vi "log analysis_gps.vi"() -> ()   [LabVIEW 2019] (continued)
,37.37108222334,126.72339800305,8.3261,22.3000,-0.1005,0.2888,0.0175,-1.549699637,0.826090686,104.570528927,0.4090,0.2977,0.5394,0.1094,0.0929,0.0762,0.1525,0.1522,4.9251,0f000001,0*19ed46e2\n\t", "INSPVAXA,USB3,0,46.5,FINESTEERING,2107,281999.350,02000000,471d,15824;INS_ALIGNMENT_COMPLETE,INS_RTKFIXED,37.37108175635,126.72339952041,8.3297,22.3000,-0.1125,0.3020,0.0389,-1.388953063,0.939960250,105.504121807,0.4075,0.2973,0.5375,0.1091,0.0928,0.0761,0.1524,0.1521,4.9251,0f000001,0*0f043892\n\t", "INSPVAXA,USB3,0,46.5,FINESTEERING,2107,281999.850,02000000,471d,15824;INS_ALIGNMENT_COMPLETE,INS_RTKFIXED,37.37108126318,126.72340101598,8.3324,22.3000,-0.1208,0.2855,0.0176,-1.235609650,1.001617450,106.317928452,0.4075,0.2973,0.5375,0.1091,0.0928,0.0761,0.1524,0.1521,4.9251,0f000001,0*a366704e\n\t", "INSPVAXA,USB3,0,45.5,FINESTEERING,2107,282000.350,02000000,471d,15824;INS_ALIGNMENT_COMPLETE,INS_RTKFIXED,37.37108078810,126.72340249141,8.3350,22.3000,-0.1085,0.2765,0.0052,-1.369966017,1.132397768,106.939829870,0.4067,0.2969,0.5359,0.1090,0.0927,0.0761,0.1523,0.1521,4.9261,0f000001,0*76e4d7c9\n\t", "INSPVAXA,USB3,0,45.5,FINESTEERING,2107,282000.850,02000000,471d,15824;INS_ALIGNMENT_COMPLETE,INS_RTKFIXED,37.37108030098,126.72340396380,8.3376,22.3000,-0.1078,0.2732,0.0027,-1.376343983,1.101027936,107.303720735,0.4067,0.2969,0.5359,0.1090,0.0927,0.0761,0.1523,0.1521,4.9261,0f000001,0*d0ca4e8b\n\t", "INSPVAXA,USB3,0,48.0,FINESTEERING,2107,282001.350,02000000,471d,15824;INS_ALIGNMENT_COMPLETE,INS_RTKFIXED,37.37107981419,126.72340544381,8.3410,22.3000,-0.1015,0.2654,0.0098,-1.448342313,0.934631006,107.625890193,0.4067,0.2967,0.5346,0.1090,0.0928,0.0761,0.1522,0.1521,4.9276,0f000001,0*0452f07a\n\t", "INSPVAXA,USB3,0,48.0,FINESTEERING,2107,282001.850,02000000,471d,15824;INS_ALIGNMENT_COMPLETE,INS_RTKFIXED,37.37107932053,126.72340689230,8.3455,22.3000,-0.1081,0.2753,0.0156,-1.395073835,0.867862564,107.855111716,0.4067,0.2967,0.5346,0.1090,0.0928,0.0761,0.1522,0.1521,4.9276,0f000001,0*57502385\n\t", "INSPVAXA,USB3,0,47.5,FINESTEERING,2107,282003.350,02000000,471d,15824;INS_ALIGNMENT_COMPLETE,INS_RTKFIXED,37.37107789784,126.72341117734,8.3560,22.3000,-0.1094,0.2769,0.0199,-1.466008388,0.636532591,108.200024976,0.4065,0.2960,0.5312,0.1093,0.0930,0.0760,0.1520,0.1521,4.9306,0f000001,0*2f9a30b4\n\t", "INSPVAXA,USB3,0,47.5,FINESTEERING,2107,282003.850,02000000,471d,15824;INS_ALIGNMENT_COMPLETE,INS_RTKFIXED,37.37107739435,126.72341272898,8.3600,22.3000,-0.1006,0.2711,0.0114,-1.521008315,0.580444752,108.231718498,0.4065,0.2960,0.5312,0.1093,0.0930,0.0760,0.1520,0.1521,4.9306,0f000001,0*1b9fd745\n\t", "INSPVAXA,USB3,0,50.0,FINESTEERING,2107,282004.350,02000000,471d,15824;INS_ALIGNMENT_COMPLETE,INS_RTKFIXED,37.37107686919,126.72341426546,8.3651,22.3000,-0.1209,0.2828,0.0059,-1.390875360,0.569748446,108.156890117,0.4068,0.2963,0.5308,0.1095,0.0933,0.0761,0.1519,0.1521,4.9320,0f000001,0*3c184099\n\t", "INSPVAXA,USB3,0,51.0,FINESTEERING,2107,282005.850,02000000,471d,15824;INS_ALIGNMENT_COMPLETE,INS_RTKFIXED,37.37107540800,126.72341870261,8.3803,22.3000,-0.1004,0.2666,0.0170,-1.392102628,0.780129510,106.805722227,0.4082,0.2971,0.5322,0.1099,0.0935,0.0762,0.1518,0.1521,4.9335,0f000001,0*c4f2d669\n\t", "INSPVAXA,USB3,0,50.5,FINESTEERING,2107,282006.350,02000000,471d,15824;INS_ALIGNMENT_COMPLETE,INS_RTKFIXED,37.37107495980,126.72342017770,8.3861,22.3000,-0.1091,0.2763,0.0150,-1.313432371,0.996573808,106.046100672,0.4084,0.2972,0.5323,0.1099,0.0934,0.0763,0.1516,0.1520,4.9349,0f000001,0*72236ee9\n\t", "INSPVAXA,USB3,0,49.0,FINESTEERING,2107,282007.350,02000000,471d,15824;INS_ALIGNMENT_COMPLETE,INS_RTKFIXED,37.37107412137,126.72342315241,8.3985,22.3000,-0.0946,0.2769,0.0276,-1.358512110,1.052240106,104.351657391,0.4091,0.2973,0.5323,0.1098,0.0932,0.0763,0.1515,0.1519,4.9361,0f000001,0*6aff20b9\n\t", "INSPVAXA,USB3,0,47.0,FINESTEERING,2107,282009.350,02000000,471d,15824;INS_ALIGNMENT_COMPLETE,INS_RTKFIXED,37.37107260212,126.72342930936,8.4118,22.3000,-0.0884,0.2755,0.0223,-1.652819508,0.448050355,102.238648457,0.4104,0.2979,0.5346,0.1094,0.0930,0.0765,0.1512,0.1518,4.9380,0f000001,0*2e51505f\n\t", "INSPVAXA,USB3,0,47.0,FINESTEERING,2107,282009.850,02000000,471d,15824;INS_ALIGNMENT_COMPLETE,INS_RTKFIXED,37.37107223648,126.72343083952,8.4130,22.3000,-0.0862,0.2839,0.0131,-1.656636551,0.434054933,102.188097613,0.4104,0.2979,0.5346,0.1094,0.0930,0.0765,0.1512,0.1518,4.9380,0f000001,0*992372f4\n\t", "INSPVAXA,USB3,0,46.0,FINESTEERING,2107,282010.350,02000000,471d,15824;INS_ALIGNMENT_COMPLETE,INS_RTKFIXED,37.37107186775,126.72343236378,8.4152,22.3000,-0.0921,0.2683,0.0190,-1.511067281,0.481994622,102.142666478,0.4105,0.2980,0.5358,0.1093,0.0929,0.0765,0.1512,0.1517,4.9389,0f000001,0*34dbbab6\n\t", "INSPVAXA,USB3,0,49.0,FINESTEERING,2107,282011.350,02000000,471d,15824;INS_ALIGNMENT_COMPLETE,INS_RTKFIXED,37.37107115288,126.72343536297,8.4170,22.3000,-0.0915,0.2655,0.0124,-1.290050138,0.612762474,102.317244842,0.4100,0.2979,0.5362,0.1091,0.0927,0.0765,0.1511,0.1517,4.9398,0f000001,0*277eff4c\n\t", "INSPVAXA,USB3,0,48.5,FINESTEERING,2107,282012.350,02000000,471d,15824;INS_ALIGNMENT_COMPLETE,INS_RTKFIXED,37.37107045869,126.72343838460,8.4146,22.3000,-0.0891,0.2830,0.0038,-1.422267126,0.594621052,102.638304107,0.4097,0.2976,0.5361,0.1090,0.0927,0.0765,0.1511,0.1517,4.9408,0f000001,0*744e9f55\n\t", "INSPVAXA,USB3,0,46.5,FINESTEERING,2107,282015.850,02000000,471d,15824;INS_ALIGNMENT_COMPLETE,INS_RTKFIXED,37.37106760969,126.72344937900,8.4187,22.3000,-0.0917,0.2780,0.0158,-0.823777305,0.513346415,106.387079923,0.4071,0.2967,0.5334,0.1088,0.0928,0.0762,0.1512,0.1516,4.9449,0f000001,0*de85c605\n\t", "INSPVAXA,USB3,0,46.0,FINESTEERING,2107,282016.350,02000000,471d,15824;INS_ALIGNMENT_COMPLETE,INS_RTKFIXED,37.37106713807,126.72345092537,8.4175,22.3000,-0.1003,0.2625,0.0249,-0.751765663,0.448430212,107.196344846,0.4062,0.2963,0.5317,0.1087,0.0929,0.0761,0.1512,0.1516,4.9459,0f000001,0*2521d5ac\n\t", "INSPVAXA,USB3,0,46.0,FINESTEERING,2107,282016.850,02000000,471d,15824;INS_ALIGNMENT_COMPLETE,INS_RTKFIXED,37.37106663656,126.72345246324,8.4162,22.3000,-0.1297,0.2604,0.0145,-0.574430267,0.261467814,108.063333899,0.4062,0.2963,0.5317,0.1087,0.0929,0.0761,0.1512,0.1516,4.9459,0f000001,0*0cb415b8\n\t", "INSPVAXA,USB3,0,49.0,FINESTEERING,2107,282026.900,02000000,471d,15824;INS_ALIGNMENT_COMPLETE,INS_RTKFIXED,37.37105597447,126.72348196925,8.3886,22.3000,-0.1101,0.2823,-0.0032,0.311492548,-0.004113518,106.939400218,0.4050,0.2960,0.5269,0.1087,0.0927,0.0760,0.1504,0.1513,4.9517,0f000001,0*e3da5464\n\t", "INSPVAXA,USB3,0,48.5,FINESTEERING,2107,282028.900,02000000,471d,15824;INS_ALIGNMENT_COMPLETE,INS_RTKFIXED,37.37105423586,126.72348799189,8.3853,22.3000,-0.0954,0.2609,0.0063,0.345591384,-0.136100185,106.270510244,0.4039,0.2954,0.5254,0.1083,0.0924,0.0759,0.1502,0.1513,4.9544,0f000001,0*0554cafd\n\t", "INSPVAXA,USB3,0,51.5,FINESTEERING,2107,282029.400,02000000,471d,15824;INS_ALIGNMENT_COMPLETE,INS_RTKFIXED,37.37105381452,126.72348943964,8.3855,22.3000,-0.0956,0.2580,0.0057,0.437004372,-0.047146220,106.316911709,0.4029,0.2951,0.5243,0.1082,0.0924,0.0758,0.1501,0.1513,4.9556,0f000001,0*8a2f1e39\n\t", "INSPVAXA,USB3,0,49.5,FINESTEERING,2107,282032.400,02000000,471d,15824;INS_ALIGNMENT_COMPLETE,INS_RTKFIXED,37.37105111138,126.72349854734,8.3925,22.3000,-0.1007,0.2882,0.0025,0.307227666,0.473154463,107.541908960,0.4011,0.2941,0.5198,0.1079,0.0924,0.0756,0.1501,0.1513,4.9577,0f000001,0*dbe53f25\n\t", "INSPVAXA,USB3,0,50.0,FINESTEERING,2107,282033.400,02008000,471d,15824;INS_ALIGNMENT_COMPLETE,INS_RTKFIXED,37.37105012658,126.72350166762,8.4012,22.3000,-0.1057,0.2825,0.0064,0.046728519,0.492534824,108.559226244,0.4006,0.2938,0.5182,0.1078,0.0924,0.0755,0.1501,0.1512,4.9578,0f000001,0*3bd3df90\n\t", "INSPVAXA,USB3,0,50.0,FINESTEERING,2107,282033.900,02008000,471d,15824;INS_ALIGNMENT_COMPLETE,INS_RTKFIXED,37.37104960391,126.72350321994,8.4050,22.3000,-0.1156,0.2745,0.0097,0.015907780,0.376843772,109.332052646,0.4006,0.2938,0.5182,0.1078,0.0924,0.0755,0.1501,0.1512,4.9578,0f000001,0*2158b20c\n\t", "INSPVAXA,USB3,0,47.5,FINESTEERING,2107,282034.400,02008000,471d,15824;INS_ALIGNMENT_COMPLETE,INS_RTKFIXED,37.37104906846,126.72350474212,8.4070,22.3000,-0.1192,0.2804,0.0105,-0.067520061,0.436867001,110.176313539,0.4000,0.2937,0.5167,0.1078,0.0924,0.0754,0.1502,0.1512,4.9578,0f000001,0*936b6da1\n\t", "INSPVAXA,USB3,0,48.0,FINESTEERING,2107,282035.400,02008000,471d,15824;INS_ALIGNMENT_COMPLETE,INS_RTKFIXED,37.37104794270,126.72350775630,8.4115,22.3000,-0.1276,0.2808,0.0020,-0.201006751,0.469956354,111.990081929,0.3992,0.2935,0.5154,0.1077,0.0923,0.0754,0.1502,0.1511,4.9577,0f000001,0*ad6b63a0\n\t", "INSPVAXA,USB3,0,48.0,FINESTEERING,2107,282035.900,02008000,471d,15824;INS_ALIGNMENT_COMPLETE,INS_RTKFIXED,37.37104734832,126.72350923933,8.4125,22.3000,-0.1168,0.2783,-0.0124,-0.218567372,0.308742852,112.764094273,0.3992,0.2935,0.5154,0.1077,0.0923,0.0754,0.1502,0.1511,4.9577,0f000001,0*3d3cbf81\n\t", "INSPVAXA,USB3,0,50.0,FINESTEERING,2107,282036.900,02008000,471d,15824;INS_ALIGNMENT_COMPLETE,INS_RTKFIXED,37.37104611251,126.72351217399,8.4148,22.3000,-0.1294,0.2583,0.0040,-0.390769339,0.147574689,113.900095191,0.3984,0.2933,0.5139,0.1077,0.0919,0.0753,0.1502,0.1511,4.9576,0f000001,0*94857a61\n\t", "INSPVAXA,USB3,0,48.0,FINESTEERING,2107,282037.400,02000000,471d,15824;INS_ALIGNMENT_COMPLETE,INS_RTKFIXED,37.37104547793,126.72351361006,8.4177,22.3000,-0.1348,0.2688,0.0058,-0.392403190,0.136695016,114.188183924,0.3974,0.2930,0.5127,0.1077,0.0918,0.0752,0.1502,0.1510,4.9580,0f000001,0*b3a6b226\n\t", "INSPVAXA,USB3,0,48.0,FINESTEERING,2107,282037.900,02000000,471d,15824;INS_ALIGNMENT_COMPLETE,INS_RTKFIXED,37.37104482885,126.72351504265,8.4195,22.3000,-0.1327,0.2535,0.0065,-0.334026852,0.167702494,114.415099877,0.3974,0.2930,0.5127,0.1077,0.0918,0.0752,0.1502,0.1510,4.9580,0f000001,0*e3ab242e\n\t", "INSPVAXA,USB3,0,48.5,FINESTEERING,2107,282038.400,02000000,471d,15824;INS_ALIGNMENT_COMPLETE,INS_RTKFIXED,37.37104419976,126.72351643213,8.4201,22.3000,-0.1292,0.2573,0.0088,-0.447214076,0.203710277,114.641680201,0.3969,0.2929,0.5120,0.1077,0.0919,0.0752,0.1502,0.1510,4.9585,0f000001,0*5ffb5d5a\n\t", "INSPVAXA,USB3,0,48.5,FINESTEERING,2107,282038.900,02000000,471d,15824;INS_ALIGNMENT_COMPLETE,INS_RTKFIXED,37.37104355987,126.72351779908,8.4210,22.3000,-0.1397,0.2477,0.0110,-0.380183542,0.075701801,114.791210844,0.3969,0.2929,0.5120,0.1077,0.0919,0.0752,0.1502,0.1510,4.9585,0f000001,0*4f3052be\n\t", "INSPVAXA,USB3,0,49.5,FINESTEERING,2107,282039.400,02000000,471d,15824;INS_ALIGNMENT_COMPLETE,INS_RTKFIXED,37.37104291933,126.72351914927,8.4230,22.3000,-0.1461,0.2586,0.0054,-0.203449941,0.032639383,114.880489837,0.3965,0.2928,0.5114,0.1077,0.0919,0.0752,0.1501,0.1510,4.9590,0f000001,0*7f207efe\n\t", "INSPVAXA,USB3,0,49.5,FINESTEERING,2107,282039.900,02000000,471d,15824;INS_ALIGNMENT_COMPLETE,INS_RTKFIXED,37.37104224465,126.72352058384,8.4263,22.3000,-0.1547,0.2700,0.0148,-0.050110889,-0.053478733,114.971719756,0.3965,0.2928,0.5114,0.1077,0.0919,0.0752,0.1501,0.1510,4.9590,0f000001,0*a22ed322\n\t", "INSPVAXA,USB3,0,45.0,FINESTEERING,2107,282040.400,02000000,471d,15824;INS_ALIGNMENT_COMPLETE,INS_RTKFIXED,37.37104154925,126.72352205735,8.4266,22.3000,-0.1535,0.2759,0.0134,0.069839878,-0.109167571,115.012196802,0.3963,0.2927,0.5107,0.1078,0.0920,0.0752,0.1500,0.1510,4.9596,0f000001,0*a12699f2\n\t", "INSPVAXA,USB3,0,45.0,FINESTEERING,2107,282040.900,02000000,471d,15824;INS_ALIGNMENT_COMPLETE,INS_RTKFIXED,37.37104084785,126.72352353291,8.4256,22.3000,-0.1448,0.2740,0.0009,0.161796846,-0.076999668,115.007657548,0.3963,0.2927,0.5107,0.1078,0.0920,0.0752,0.1500,0.1510,4.9596,0f000001,0*3a67e90b\n\t", "INSPVAXA,USB3,0,50.0,FINESTEERING,2107,282041.400,02000000,471d,15824;INS_ALIGNMENT_COMPLETE,INS_RTKFIXED,37.37104019644,126.72352491689,8.4246,22.3000,-0.1518,0.2723,-0.0022,0.212334944,-0.070041433,114.640487697,0.3961,0.2927,0.5104,0.1077,0.0921,0.0751,0.1499,0.1510,4.9600,0f000001,0*8b513f40\n\t", "INSPVAXA,USB3,0,50.0,FINESTEERING,2107,282041.900,02000000,471d,15824;INS_ALIGNMENT_COMPLETE,INS_RTKFIXED,37.37103955120,126.72352632757,8.4231,22.3000,-0.1599,0.2675,-0.0000,0.251612681,-0.024570483,114.066468030,0.3961,0.2927,0.5104,0.1077,0.0921,0.0751,0.1499,0.1510,4.9600,0f000001,0*ee21d353\n\t", "INSPVAXA,USB3,0,49.0,FINESTEERING,2107,282043.400,02000000,471d,15824;INS_ALIGNMENT_COMPLETE,INS_RTKFIXED,37.37103775397,126.72353053671,8.4224,22.3000,-0.1356,0.2719,-0.0039,0.469507443,0.217168676,111.114657761,0.4278,0.2934,0.5225,0.1125,0.0922,0.0761,0.1498,0.1516,4.9609,0f000001,0*26bfa601\n\t", "INSPVAXA,USB3,0,49.0,FINESTEERING,2107,282043.900,02000000,471d,15824;INS_ALIGNMENT_COMPLETE,INS_RTKFIXED,37.37103719773,126.72353199656,8.4232,22.3000,-0.1151,0.2555,0.0099,0.378672959,0.355237505,110.161764009,0.4278,0.2934,0.5225,0.1125,0.0922,0.0761,0.1498,0.1516,4.9609,0f000001,0*a56cfb0a\n\t", "INSPVAXA,USB3,0,49.0,FINESTEERING,2107,282044.400,02000000,471d,15824;INS_ALIGNMENT_COMPLETE,INS_RTKFIXED,37.37103668630,126.72353343626,8.4255,22.3000,-0.1146,0.2521,0.0005,0.230484735,0.495195972,109.291973317,0.4151,0.2930,0.5192,0.1093,0.0918,0.0756,0.1496,0.1511,4.9617,0f000001,0*69c2d113\n\t", "INSPVAXA,USB3,0,49.0,FINESTEERING,2107,282044.900,02000000,471d,15824;INS_ALIGNMENT_COMPLETE,INS_RTKFIXED,37.37103618153,126.72353489391,8.4287,22.3000,-0.1231,0.2600,0.0038,0.173840708,0.566394531,108.664354090,0.4151,0.2930,0.5192,0.1093,0.0918,0.0756,0.1496,0.1511,4.9617,0f000001,0*5975ddd2\n\t", "INSPVAXA,USB3,0,50.5,FINESTEERING,2107,282045.400,02000000,471d,15824;INS_ALIGNMENT_COMPLETE,INS_RTKFIXED,37.37103569365,126.72353637102,8.4304,22.3000,-0.1241,0.2677,0.0051,0.029985100,0.713380187,108.316777088,0.4073,0.2928,0.5168,0.1078,0.0917,0.0754,0.1495,0.1510,4.9629,0f000001,0*ed89f5e7\n\t", "INSPVAXA,USB3,0,50.5,FINESTEERING,2107,282045.900,02000000,471d,15824;INS_ALIGNMENT_COMPLETE,INS_RTKFIXED,37.37103520329,126.72353786687,8.4303,22.3000,-0.1276,0.2596,0.0072,-0.128043744,0.852574922,108.131029460,0.4073,0.2928,0.5168,0.1078,0.0917,0.0754,0.1495,0.1510,4.9629,0f000001,0*d9490397\n\t", "INSPVAXA,USB3,0,47.5,FINESTEERING,2107,282046.400,02000000,471d,15824;INS_ALIGNMENT_COMPLETE,INS_RTKFIXED,37.37103472430,126.72353933486,8.4326,22.3000,-0.1274,0.2469,0.0233,-0.197512090,0.856787490,108.035575182,0.4031,0.2927,0.5152,0.1074,0.0918,0.0753,0.1494,0.1509,4.9644,0f000001,0*7594b79a\n\t", "INSPVAXA,USB3,0,47.5,FINESTEERING,2107,282046.900,02000000,471d,15824;INS_ALIGNMENT_COMPLETE,INS_RTKFIXED,37.37103423045,126.72354082894,8.4356,22.3000,-0.1317,0.2525,0.0181,-0.272615220,0.680276177,108.135899637,0.4031,0.2927,0.5152,0.1074,0.0918,0.0753,0.1494,0.1509,4.9644,0f000001,0*0ad6ca19\n\t", "INSPVAXA,USB3,0,50.0,FINESTEERING,2107,282047.400,02000000,471d,15824;INS_ALIGNMENT_COMPLETE,INS_RTKFIXED,37.37103373575,126.72354228047,8.4378,22.3000,-0.1209,0.2496,0.0116,-0.304500119,0.597497624,108.265546221,0.4007,0.2928,0.5142,0.1074,0.0918,0.0752,0.1494,0.1510,4.9658,0f000001,0*f7570865\n\t", "INSPVAXA,USB3,0,50.0,FINESTEERING,2107,282047.900,02000000,471d,15824;INS_ALIGNMENT_COMPLETE,INS_RTKFIXED,37.37103324070,126.72354372631,8.4396,22.3000,-0.1245,0.2634,0.0029,-0.432470862,0.435465093,108.449839156,0.4007,0.2928,0.5142,0.1074,0.0918,0.0752,0.1494,0.1510,4.9658,0f000001,0*36db7439\n\t", "INSPVAXA,USB3,0,50.5,FINESTEERING,2107,282048.400,02000000,471d,15824;INS_ALIGNMENT_COMPLETE,INS_RTKFIXED,37.37103276390,126.72354512195,8.4422,22.3000,-0.1174,0.2527,0.0035,-0.579219064,0.548453263,108.588640946,0.3999,0.2929,0.5136,0.1077,0.0919,0.0752,0.1494,0.1510,4.9669,0f000001,0*39dcb86d\n\t", "INSPVAXA,USB3,0,50.5,FINESTEERING,2107,282048.900,02000000,471d,15824;INS_ALIGNMENT_COMPLETE,INS_RTKFIXED,37.37103224560,126.72354663214,8.4444,22.3000,-0.1277,0.2757,0.0017,-0.626592157,0.566170063,108.836719215,0.3999,0.2929,0.5136,0.1077,0.0919,0.0752,0.1494,0.1510,4.9669,0f000001,0*2908ea23\n\t", "INSPVAXA,USB3,0,49.5,FINESTEERING,2107,282049.400,02000000,471d,15824;INS_ALIGNMENT_COMPLETE,INS_RTKFIXED,37.37103169688,126.72354817389,8.4462,22.3000,-0.1370,0.2620,0.0032,-0.416455659,0.615214543,109.052473427,0.3987,0.2929,0.5129,0.1079,0.0918,0.0751,0.1495,0.1510,4.9681,0f000001,0*9e3ef17b\n\t", "INSPVAXA,USB3,0,49.5,FINESTEERING,2107,282049.900,02000000,471d,15824;INS_ALIGNMENT_COMPLETE,INS_RTKFIXED,37.37103115870,126.72354965807,8.4484,22.3000,-0.1429,0.2729,-0.0002,-0.328473070,0.641311301,109.380425466,0.3987,0.2929,0.5129,0.1079,0.0918,0.0751,0.1495,0.1510,4.9681,0f000001,0*d7629724\n\t", "INSPVAXA,USB3,0,50.0,FINESTEERING,2107,282050.400,02000000,471d,15824;INS_ALIGNMENT_COMPLETE,INS_RTKFIXED,37.37103062705,126.72355118407,8.4512,22.3000,-0.1472,0.2693,0.0005,-0.421432718,0.551827258,109.755848199,0.3977,0.2928,0.5121,0.1079,0.0919,0.0751,0.1495,0.1509,4.9692,0f000001,0*9b0507cc\n\t", "INSPVAXA,USB3,0,50.0,FINESTEERING,2107,282050.900,02000000,471d,15824;INS_ALIGNMENT_COMPLETE,INS_RTKFIXED,37.37103009197,126.72355271256,8.4539,22.3000,-0.1417,0.2757,0.0094,-0.635318550,0.518176153,110.294243776,0.3977,0.2928,0.5121,0.1079,0.0919,0.0751,0.1495,0.1509,4.9692,0f000001,0*281a41b6\n\t", "INSPVAXA,USB3,0,48.0,FINESTEERING,2107,282051.400,02000000,471d,15824;INS_ALIGNMENT_COMPLETE,INS_RTKFIXED,37.37102952977,126.72355418303,8.4573,22.3000,-0.1452,0.2608,-0.0009,-0.446409440,0.466780038,110.936496346,0.3976,0.2929,0.5117,0.1080,0.0918,0.0751,0.1495,0.1509,4.9703,0f000001,0*e106e6fe\n\t", "INSPVAXA,USB3,0,48.0,FINESTEERING,2107,282051.900,02000000,471d,15824;INS_ALIGNMENT_COMPLETE,INS_RTKFIXED,37.37102892561,126.72355566978,8.4607,22.3000,-0.1442,0.2601,0.0120,-0.193968959,0.359112496,111.726524346,0.3976,0.2929,0.5117,0.1080,0.0918,0.0751,0.1495,0.1509,4.9703,0f000001,0*bd701264\n\t", "INSPVAXA,USB3,0,46.5,FINESTEERING,2107,282052.400,02000000,471d,15824;INS_ALIGNMENT_COMPLETE,INS_RTKFIXED,37.37102834660,126.72355712345,8.4631,22.3000,-0.1344,0.2420,0.0090,-0.254926417,0.436150918,112.550580060,0.3973,0.2929,0.5110,0.1078,0.0918,0.0751,0.1495,0.1508,4.9714,0f000001,0*49726e9c\n\t", "INSPVAXA,USB3,0,46.5,FINESTEERING,2107,282052.900,02000000,471d,15824;INS_ALIGNMENT_COMPLETE,INS_RTKFIXED,37.37102775131,126.72355855890,8.4646,22.3000,-0.1511,0.2448,0.0254,-0.250642756,0.477147225,113.358906308,0.3973,0.2929,0.5110,0.1078,0.0918,0.0751,0.1495,0.1508,4.9714,0f000001,0*ce9979aa\n\t", "INSPVAXA,USB3,0,44.5,FINESTEERING,2107,282053.400,02000000,471d,15824;INS_ALIGNMENT_COMPLETE,INS_RTKFIXED,37.37102714809,126.72355999231,8.4667,22.3000,-0.1605,0.2545,0.0109,-0.233782899,0.571505620,114.141889462,0.3971,0.2928,0.5106,0.1077,0.0917,0.0750,0.1495,0.1507,4.9724,0f000001,0*6bed7872\n\t", "DUALANTENNAHEADINGA,USB3,0,44.5,FINESTEERING,2107,282053.900,02000000,d426,15824;SOL_COMPUTED,NARROW_FLOAT,-1.000000000,165.380935669,31.219970703,0.0,261.390197754,180.000000000,\"631T\",19,7,7,7,04,00,20,03*4f993fc4\n\t", "INSPVAXA,USB3,0,48.0,FINESTEERING,2107,282054.400,02000000,471d,15824;INS_ALIGNMENT_COMPLETE,INS_RTKFIXED,37.37102588447,126.72356281881,8.4708,22.3000,-0.1681,0.2698,0.0199,0.211462800,0.565070170,115.259101386,0.3974,0.2928,0.5104,0.1076,0.0917,0.0751,0.1495,0.1506,4.9735,0f000001,0*fe4062de\n\t", "INSPVAXA,USB3,0,48.0,FINESTEERING,2107,282054.900,02000000,471d,15824;INS_ALIGNMENT_COMPLETE,INS_RTKFIXED,37.37102524848,126.72356421796,8.4709,22.3000,-0.1622,0.2530,-0.0006,0.102305423,0.525752233,115.651365939,0.3974,0.2928,0.5104,0.1076,0.0917,0.0751,0.1495,0.1506,4.9735,0f000001,0*0e3012d6\n\t", "INSPVAXA,USB3,0,46.5,FINESTEERING,2107,282055.400,02000000,471d,15824;INS_ALIGNMENT_COMPLETE,INS_RTKFIXED,37.37102459483,126.72356562736,8.4700,22.3000,-0.1625,0.2569,-0.0075,0.070588481,0.412699361,115.906103651,0.4155,0.2932,0.5168,0.1107,0.0919,0.0756,0.1495,0.1510,4.9747,0f000001,0*738f8c7d\n\t", "INSPVAXA,USB3,0,46.5,FINESTEERING,2107,282055.900,02000000,471d,15824;INS_ALIGNMENT_COMPLETE,INS_RTKFIXED,37.37102394338,126.72356697461,8.4688,22.3000,-0.1600,0.2462,-0.0061,0.217668333,0.474174872,116.134195625,0.4155,0.2932,0.5168,0.1107,0.0919,0.0756,0.1495,0.1510,4.9747,0f000001,0*22c3b36b\n\t", "INSPVAXA,USB3,0,48.0,FINESTEERING,2107,282056.400,02000000,471d,15824;INS_ALIGNMENT_COMPLETE,INS_RTKFIXED,37.37102326974,126.72356835081,8.4675,22.3000,-0.1698,0.2576,-0.0043,0.387693340,0.353581686,116.290488152,0.4308,0.2936,0.5243,0.1128,0.0921,0.0761,0.1495,0.1513,4.9761,0f000001,0*4bf67f5e\n\t", "DUALANTENNAHEADINGA,USB3,0,48.0,FINESTEERING,2107,282056.900,02000000,d426,15824;SOL_COMPUTED,L1_FLOAT,-1.000000000,188.034057617,48.521991730,0.0,149.833007813,180.000000000,\"631T\",17,7,7,7,04,00,20,03*4a1bc78c\n\t", "INSPVAXA,USB3,0,49.5,FINESTEERING,2107,282057.400,02000000,471d,15824;INS_ALIGNMENT_COMPLETE,INS_RTKFIXED,37.37102198176,126.72357104397,8.4666,22.3000,-0.1730,0.2276,-0.0046,0.296246592,0.281453997,116.587848153,0.4169,0.2930,0.5203,0.1094,0.0919,0.0756,0.1494,0.1507,4.9775,0f000001,0*365c3542\n\t", "INSPVAXA,USB3,0,49.5,FINESTEERING,2107,282057.900,02000000,471d,15824;INS_ALIGNMENT_COMPLETE,INS_RTKFIXED,37.37102132674,126.72357243204,8.4681,22.3000,-0.1784,0.2359,-0.0022,0.276182941,0.305119300,116.637377638,0.4169,0.2930,0.5203,0.1094,0.0919,0.0756,0.1494,0.1507,4.9775,0f000001,0*2cc7c943\n\t", "INSPVAXA,USB3,0,46.0,FINESTEERING,2107,282058.400,02000000,471d,15824;INS_ALIGNMENT_COMPLETE,INS_RTKFIXED,37.37102064028,126.72357384993,8.4690,22.3000,-0.1826,0.2708,0.0015,0.277724893,0.355072296,116.706780756,0.4085,0.2927,0.5173,0.1080,0.0919,0.0753,0.1493,0.1505,4.9788,0f000001,0*091434dc\n\t", "DUALANTENNAHEADINGA,USB3,0,46.0,FINESTEERING,2107,282058.900,02000000,d426,15824;SOL_COMPUTED,NARROW_FLOAT,-1.000000000,155.425567627,41.921077728,0.0,360.000000000,180.000000000,\"631T\",17,7,7,7,04,00,20,03*1ade94fd\n\t", "DUALANTENNAHEADINGA,USB3,0,47.5,FINESTEERING,2107,282059.400,02000000,d426,15824;SOL_COMPUTED,NARROW_FLOAT,-1.000000000,183.622436523,40.173770905,0.0,305.777679443,180.000000000,\"631T\",17,7,7,7,04,00,20,03*be7303c1\n\t", "DUALANTENNAHEADINGA,USB3,0,47.5,FINESTEERING,2107,282059.900,02000000,d426,15824;SOL_COMPUTED,NARROW_FLOAT,-1.000000000,183.595245361,41.079216003,0.0,306.083618164,180.000000000,\"631T\",17,7,7,7,04,00,20,02*56ca6491\n\t", "DUALANTENNAHEADINGA,USB3,0,50.5,FINESTEERING,2107,282060.400,02000000,d426,15824;SOL_COMPUTED,L1_FLOAT,-1.000000000,188.621459961,32.809661865,0.0,201.470733643,180.000000000,\"631T\",16,6,6,6,04,00,20,02*4c9b8a65\n\t", "DUALANTENNAHEADINGA,USB3,0,50.5,FINESTEERING,2107,282060.900,02000000,d426,15824;SOL_COMPUTED,L1_FLOAT,-1.000000000,188.468612671,32.503238678,0.0,203.530487061,180.000000000,\"631T\",16,6,6,6,04,00,20,02*a42a0267\n\t", "INSPVAXA,USB3,0,52.0,FINESTEERING,2107,282061.400,02000000,471d,15824;INS_ALIGNMENT_COMPLETE,INS_RTKFIXED,37.37101652600,126.72358236543,8.4736,22.3000,-0.1613,0.2499,-0.0018,0.130104122,0.184346259,115.264963296,0.3994,0.2931,0.5137,0.1077,0.0920,0.0751,0.1491,0.1505,4.9829,0f000001,0*84f4c641\n\t", "INSPVAXA,USB3,0,52.0,FINESTEERING,2107,282061.900,02000000,471d,15824;INS_ALIGNMENT_COMPLETE,INS_RTKFIXED,37.37101586728,126.72358376934,8.4724,22.3000,-0.1591,0.2551,-0.0023,0.208355260,0.306813184,114.636507713,0.3994,0.2931,0.5137,0.1077,0.0920,0.0751,0.1491,0.1505,4.9829,0f000001,0*6df399da\n\t", "DUALANTENNAHEADINGA,USB3,0,49.0,FINESTEERING,2107,282062.400,02000000,d426,15824;SOL_COMPUTED,NARROW_FLOAT,-1.000000000,152.663146973,-31.160461426,0.0,360.000000000,180.000000000,\"631T\",16,6,6,6,04,00,20,03*79a87a98\n\t", "INSPVAXA,USB3,0,49.0,FINESTEERING,2107,282062.900,02000000,471d,15824;INS_ALIGNMENT_COMPLETE,INS_RTKFIXED,37.37101460250,126.72358663230,8.4657,22.3000,-0.1655,0.2464,-0.0060,0.173361139,0.049133885,113.278518772,0.3984,0.2930,0.5124,0.1078,0.0919,0.0750,0.1489,0.1506,4.9845,0f000001,0*56ff342f\n\t", "INSPVAXA,USB3,0,50.0,FINESTEERING,2107,282063.400,02000000,471d,15824;INS_ALIGNMENT_COMPLETE,INS_RTKFIXED,37.37101399789,126.72358807716,8.4654,22.3000,-0.1571,0.2332,0.0025,0.071973073,0.119158160,112.739398614,0.3982,0.2929,0.5114,0.1079,0.0918,0.0750,0.1488,0.1506,4.9861,0f000001,0*f4c7a0fa\n\t", "DUALANTENNAHEADINGA,USB3,0,50.0,FINESTEERING,2107,282063.900,02000000,d426,15824;SOL_COMPUTED,NARROW_FLOAT,-1.000000000,151.658050537,-47.108062744,0.0,360.000000000,180.000000000,\"631T\",15,6,6,6,04,00,20,03*1e02ddce\n\t", "INSPVAXA,USB3,0,49.5,FINESTEERING,2107,282064.400,02008000,471d,15824;INS_ALIGNMENT_COMPLETE,INS_RTKFIXED,37.37101278897,126.72359100387,8.4654,22.3000,-0.1602,0.2656,-0.0115,0.293522321,0.241172864,111.956840334,0.3974,0.2927,0.5103,0.1078,0.0917,0.0750,0.1488,0.1506,4.9877,0f000001,0*fae7c97d\n\t", "DUALANTENNAHEADINGA,USB3,0,49.5,FINESTEERING,2107,282064.900,02008000,d426,15824;SOL_COMPUTED,NARROW_FLOAT,-1.000000000,152.203399658,-59.519470215,0.0,360.000000000,180.000000000,\"631T\",18,7,7,6,04,00,20,03*8e7f9ac2\n\t", "DUALANTENNAHEADINGA,USB3,0,49.5,FINESTEERING,2107,282065.400,02008000,d426,15824;SOL_COMPUTED,NARROW_FLOAT,-1.000000000,122.017272949,78.944664001,0.0,360.000000000,167.907485962,\"631T\",17,7,7,7,04,00,20,03*05083127\n\t", "DUALANTENNAHEADINGA,USB3,0,49.5,FINESTEERING,2107,282065.900,02008000,d426,15824;SOL_COMPUTED,NARROW_FLOAT,-1.000000000,121.918090820,78.941169739,0.0,360.000000000,169.045944214,\"631T\",18,7,7,7,04,00,20,03*3f11d063\n\t", "DUALANTENNAHEADINGA,USB3,0,48.0,FINESTEERING,2107,282066.400,02008000,d426,15824;SOL_COMPUTED,NARROW_FLOAT,-1.000000000,150.971466064,30.315032959,0.0,360.000000000,180.000000000,\"631T\",21,7,7,7,04,00,20,03*10224658\n\t", "DUALANTENNAHEADINGA,USB3,0,48.0,FINESTEERING,2107,282066.900,02008000,d426,15824;SOL_COMPUTED,NARROW_FLOAT,-1.000000000,150.582351685,29.219997406,0.0,360.000000000,180.000000000,\"631T\",21,7,7,7,04,00,20,03*814dc40f\n\t", "DUALANTENNAHEADINGA,USB3,0,50.0,FINESTEERING,2107,282067.400,02008000,d426,15824;SOL_COMPUTED,NARROW_FLOAT,-1.000000000,145.294387817,24.460121155,0.0,360.000000000,180.000000000,\"631T\",20,7,7,7,04,00,20,03*8bfd9c96\n\t", "DUALANTENNAHEADINGA,USB3,0,50.0,FINESTEERING,2107,282067.900,02008000,d426,15824;SOL_COMPUTED,NARROW_FLOAT,-1.000000000,143.647583008,28.839637756,0.0,360.000000000,180.000000000,\"631T\",18,7,7,7,04,00,20,03*4514f4b2\n\t", "INSPVAXA,USB3,0,47.0,FINESTEERING,2107,282068.400,02000000,471d,15824;INS_ALIGNMENT_COMPLETE,INS_RTKFIXED,37.37100819818,126.72360279226,8.4607,22.3000,-0.1621,0.2796,-0.0079,-0.283387467,0.022264293,112.218267949,0.3978,0.2926,0.5089,0.1077,0.0918,0.0750,0.1487,0.1505,4.9920,0f000001,0*2b60bbde\n\t", "DUALANTENNAHEADINGA,USB3,0,47.0,FINESTEERING,2107,282068.900,02000000,d426,15824;SOL_COMPUTED,NARROW_FLOAT,-1.000000000,100.644241333,68.634323120,0.0,360.000000000,124.100311279,\"631T\",21,7,7,7,04,00,20,03*c3cc83cc\n\t", "DUALANTENNAHEADINGA,USB3,0,46.5,FINESTEERING,2107,282069.400,02000000,d426,15824;SOL_COMPUTED,NARROW_FLOAT,-1.000000000,62.887535095,72.941581726,0.0,329.144042969,92.146186829,\"631T\",20,7,7,7,04,00,20,03*4ebf539f\n\t", "DUALANTENNAHEADINGA,USB3,0,46.5,FINESTEERING,2107,282069.900,02000000,d426,15824;SOL_COMPUTED,NARROW_FLOAT,-1.000000000,62.622955322,73.006401062,0.0,328.499725342,92.030387878,\"631T\",20,7,7,7,04,00,20,03*db3abc9d\n\t", "DUALANTENNAHEADINGA,USB3,0,42.0,FINESTEERING,2107,282070.400,02008000,d426,15824;SOL_COMPUTED,NARROW_FLOAT,-1.000000000,164.998916626,60.444377899,0.0,329.796081543,180.000000000,\"631T\",21,7,7,7,04,00,20,03*8640d9ed\n\t", "DUALANTENNAHEADINGA,USB3,0,42.0,FINESTEERING,2107,282070.900,02008000,d426,15824;SOL_COMPUTED,NARROW_FLOAT,-1.000000000,166.059432983,59.466281891,0.0,316.536041260,180.000000000,\"631T\",22,7,7,7,04,00,20,03*a557aca2\n\t", "DUALANTENNAHEADINGA,USB3,0,47.0,FINESTEERING,2107,282071.400,02008000,d426,15824;SOL_COMPUTED,NARROW_FLOAT,-1.000000000,165.423980713,-15.767028809,0.0,239.021484375,180.000000000,\"631T\",20,7,7,7,04,00,20,03*cfd53cf7\n\t", "DUALANTENNAHEADINGA,USB3,0,47.0,FINESTEERING,2107,282071.900,02008000,d426,15824;SOL_COMPUTED,NARROW_FLOAT,-1.000000000,165.887359619,-16.480316162,0.0,236.674011230,180.000000000,\"631T\",20,7,7,7,04,00,20,03*dd935a36\n\t", "DUALANTENNAHEADINGA,USB3,0,49.5,FINESTEERING,2107,282072.400,02008000,d426,15824;SOL_COMPUTED,NARROW_FLOAT,-1.000000000,175.843307495,41.730823517,0.0,200.143447876,180.000000000,\"631T\",21,7,7,7,04,00,20,03*fbe9d2f7\n\t", "DUALANTENNAHEADINGA,USB3,0,49.5,FINESTEERING,2107,282072.900,02008000,d426,15824;SOL_COMPUTED,NARROW_FLOAT,-1.000000000,175.657180786,43.295608521,0.0,201.745788574,180.000000000,\"631T\",21,7,7,7,04,00,20,03*de4c8f7d\n\t", "DUALANTENNAHEADINGA,USB3,0,50.0,FINESTEERING,2107,282073.400,02008000,d426,15824;SOL_COMPUTED,NARROW_FLOAT,-1.000000000,88.259048462,72.880012512,0.0,360.000000000,91.084091187,\"631T\",19,7,7,7,04,00,20,03*7543b6a9\n\t", "DUALANTENNAHEADINGA,USB3,0,48.5,FINESTEERING,2107,282074.400,02000000,d426,15824;SOL_COMPUTED,NARROW_FLOAT,-1.000000000,187.625686646,-11.833007813,0.0,215.399688721,180.000000000,\"631T\",19,7,7,7,04,00,20,03*14c71104\n\t", "DUALANTENNAHEADINGA,USB3,0,49.5,FINESTEERING,2107,282075.400,02000000,d426,15824;SOL_COMPUTED,L1_FLOAT,-1.000000000,190.728332520,52.272701263,0.0,209.958755493,180.000000000,\"631T\",21,7,7,7,04,00,20,02*2a740797\n\t", "DUALANTENNAHEADINGA,USB3,0,49.5,FINESTEERING,2107,282075.900,02000000,d426,15824;SOL_COMPUTED,L1_FLOAT,-1.000000000,190.868621826,51.534015656,0.0,206.683425903,180.000000000,\"631T\",14,7,7,7,04,00,20,03*060951e8\n\t", "DUALANTENNAHEADINGA,USB3,0,44.0,FINESTEERING,2107,282076.400,02000000,d426,15824;SOL_COMPUTED,NARROW_FLOAT,-1.000000000,164.765243530,-0.145935059,0.0,360.000000000,180.000000000,\"631T\",15,7,7,7,04,00,20,03*df327d6c\n\t", "DUALANTENNAHEADINGA,USB3,0,48.0,FINESTEERING,2107,282077.900,02000000,d426,15824;SOL_COMPUTED,NARROW_FLOAT,-1.000000000,163.219406128,-2.743896484,0.0,360.000000000,180.000000000,\"631T\",17,7,7,7,04,00,20,03*74221424\n\t", "DUALANTENNAHEADINGA,USB3,0,48.5,FINESTEERING,2107,282078.400,02000000,d426,15824;SOL_COMPUTED,NARROW_FLOAT,-1.000000000,164.756866455,-2.259979248,0.0,360.000000000,180.000000000,\"631T\",19,7,7,7,04,00,20,03*e2d4ab8a\n\t", "DUALANTENNAHEADINGA,USB3,0,48.5,FINESTEERING,2107,282078.900,02000000,d426,15824;SOL_COMPUTED,NARROW_FLOAT,-1.000000000,165.064834595,-2.246643066,0.0,360.000000000,180.000000000,\"631T\",18,7,7,7,04,00,20,03*e6e75529\n\t", "DUALANTENNAHEADINGA,USB3,0,47.5,FINESTEERING,2107,282079.400,02000000,d426,15824;SOL_COMPUTED,NARROW_FLOAT,-1.000000000,174.896926880,-30.356231689,0.0,360.000000000,180.000000000,\"631T\",18,7,7,7,04,00,20,03*d638673a\n\t", "DUALANTENNAHEADINGA,USB3,0,47.5,FINESTEERING,2107,282079.900,02000000,d426,15824;SOL_COMPUTED,NARROW_FLOAT,-1.000000000,174.578781128,-31.075134277,0.0,360.000000000,180.000000000,\"631T\",17,7,7,7,04,00,20,03*d8acf742\n\t", "DUALANTENNAHEADINGA,USB3,0,48.5,FINESTEERING,2107,282081.400,02000000,d426,15824;SOL_COMPUTED,NARROW_FLOAT,-1.000000000,186.002395630,72.538307190,0.0,360.000000000,180.000000000,\"631T\",18,7,7,7,04,00,20,02*94d40da5\n\t", "INSPVAXA,USB3,0,48.0,FINESTEERING,2107,282083.450,02000000,471d,15824;INS_ALIGNMENT_COMPLETE,INS_RTKFIXED,37.37098848557,126.72364391635,8.5085,22.3000,-0.1545,0.2353,-0.0017,0.125081225,0.334802471,116.544491320,0.3966,0.2931,0.5085,0.1074,0.0919,0.0749,0.1481,0.1501,5.0097,0f000001,0*707b4fda\n\t", "INSPVAXA,USB3,0,48.0,FINESTEERING,2107,282083.950,02000000,471d,15824;INS_ALIGNMENT_COMPLETE,INS_RTKFIXED,37.37098781334,126.72364531945,8.5061,22.3000,-0.1397,0.2470,-0.0039,0.130744788,0.168821644,116.045699984,0.3966,0.2931,0.5085,0.1074,0.0919,0.0749,0.1481,0.1501,5.0097,0f000001,0*8c7cd4e3\n\t", "INSPVAXA,USB3,0,49.5,FINESTEERING,2107,282084.450,02000000,471d,15824;INS_ALIGNMENT_COMPLETE,INS_RTKFIXED,37.37098717814,126.72364671785,8.5044,22.3000,-0.1354,0.2435,-0.0138,-0.054756889,-0.022563669,115.524105800,0.3967,0.2930,0.5082,0.1073,0.0917,0.0749,0.1480,0.1501,5.0101,0f000001,0*e14fe85b\n\t", "DUALANTENNAHEADINGA,USB3,0,49.5,FINESTEERING,2107,282084.900,02000000,d426,15824;SOL_COMPUTED,NARROW_FLOAT,-1.000000000,161.093994141,-39.642028809,0.0,360.000000000,180.000000000,\"631T\",18,7,7,7,04,00,20,02*551afc73\n\t", "INSPVAXA,USB3,0,45.5,FINESTEERING,2107,282086.950,02000000,471d,15824;INS_ALIGNMENT_COMPLETE,INS_RTKFIXED,37.37098400291,126.72365390857,8.5011,22.3000,-0.1413,0.2614,-0.0071,-0.222662760,-0.431667529,114.703885924,0.3961,0.2927,0.5077,0.1073,0.0916,0.0749,0.1479,0.1501,5.0112,0f000001,0*8c0cd5e8\n\t", "INSPVAXA,USB3,0,49.0,FINESTEERING,2107,282087.950,02000000,471d,15824;INS_ALIGNMENT_COMPLETE,INS_RTKFIXED,37.37098277282,126.72365670812,8.5043,22.3000,-0.1437,0.2560,-0.0135,-0.068385407,-0.323416769,114.901118705,0.3958,0.2926,0.5076,0.1072,0.0916,0.0749,0.1479,0.1502,5.0118,0f000001,0*c54dad40\n\t", "INSPVAXA,USB3,0,45.0,FINESTEERING,2107,282088.450,02000000,471d,15824;INS_ALIGNMENT_COMPLETE,INS_RTKFIXED,37.37098213793,126.72365811830,8.5048,22.3000,-0.1404,0.2509,-0.0150,-0.140571199,-0.324537767,115.053900448,0.3958,0.2925,0.5075,0.1072,0.0917,0.0749,0.1479,0.1502,5.0126,0f000001,0*5d76f850\n\t", "INSPVAXA,USB3,0,50.0,FINESTEERING,2107,282089.950,02000000,471d,15824;INS_ALIGNMENT_COMPLETE,INS_RTKFIXED,37.37098017514,126.72366234895,8.5129,22.3000,-0.1403,0.2638,-0.0115,0.068877400,-0.331025917,115.512688537,0.3958,0.2925,0.5074,0.1072,0.0917,0.0749,0.1479,0.1501,5.0134,0f000001,0*45d8cdd7\n\t", "INSPVAXA,USB3,0,47.0,FINESTEERING,2107,282090.450,02000000,471d,15824;INS_ALIGNMENT_COMPLETE,INS_RTKFIXED,37.37097950653,126.72366381280,8.5149,22.3000,-0.1497,0.2592,-0.0041,-0.040058431,-0.070783873,115.696569109,0.3958,0.2925,0.5072,0.1072,0.0918,0.0748,0.1480,0.1501,5.0142,0f000001,0*06fd62fb\n\t", "DUALANTENNAHEADINGA,USB3,0,47.0,FINESTEERING,2107,282090.900,02000000,d426,15824;SOL_COMPUTED,NARROW_FLOAT,-1.000000000,171.721908569,34.681911469,0.0,360.000000000,180.000000000,\"631T\",20,7,7,7,04,00,20,03*da0d38e5\n\t", "INSPVAXA,USB3,0,47.0,FINESTEERING,2107,282091.450,02000000,471d,15824;INS_ALIGNMENT_COMPLETE,INS_RTKFIXED,37.37097820755,126.72366660545,8.5215,22.3000,-0.1497,0.2548,0.0005,-0.143132038,0.926627328,116.158649383,0.3959,0.2925,0.5072,0.1072,0.0918,0.0748,0.1480,0.1501,5.0152,0f000001,0*c99bd82f\n\t", "DUALANTENNAHEADINGA,USB3,0,47.0,FINESTEERING,2107,282091.900,02000000,d426,15824;SOL_COMPUTED,NARROW_FLOAT,-1.000000000,112.916130066,31.135679245,0.0,360.000000000,180.000000000,\"631T\",17,8,8,7,04,00,20,03*e78407cb\n\t", "INSPVAXA,USB3,0,44.5,FINESTEERING,2107,282092.950,02000000,471d,15824;INS_ALIGNMENT_COMPLETE,INS_RTKFIXED,37.37097614467,126.72367094542,8.5349,22.3000,-0.1554,0.2816,0.0034,-0.093672408,0.920148848,117.196010792,0.3968,0.2926,0.5073,0.1073,0.0918,0.0749,0.1480,0.1500,5.0167,0f000001,0*78c5bf02\n\t", "INSPVAXA,USB3,0,49.0,FINESTEERING,2107,282093.450,02000000,471d,15824;INS_ALIGNMENT_COMPLETE,INS_RTKFIXED,37.37097543650,126.72367235664,8.5399,22.3000,-0.1638,0.2823,0.0033,-0.126887111,0.570236621,117.700862791,0.3975,0.2926,0.5072,0.1072,0.0917,0.0749,0.1480,0.1500,5.0184,0f000001,0*ead874db\n\t", "DUALANTENNAHEADINGA,USB3,0,49.0,FINESTEERING,2107,282093.900,02000000,d426,15824;SOL_COMPUTED,NARROW_FLOAT,-1.000000000,156.493606567,-47.281768799,0.0,360.000000000,180.000000000,\"631T\",19,7,7,7,04,00,20,03*77a80aac\n\t", "INSPVAXA,USB3,0,47.0,FINESTEERING,2107,282096.950,02000000,471d,15824;INS_ALIGNMENT_COMPLETE,INS_RTKFIXED,37.37097045983,126.72368185203,8.5832,22.3000,-0.1608,0.2476,0.0236,-0.099484529,1.317134321,120.192875691,0.3973,0.2927,0.5071,0.1071,0.0916,0.0748,0.1480,0.1498,5.0232,0f000001,0*5f8f6166\n\t", "INSPVAXA,USB3,0,49.5,FINESTEERING,2107,282097.450,02000000,471d,15824;INS_ALIGNMENT_COMPLETE,INS_RTKFIXED,37.37096974645,126.72368313135,8.5891,22.3000,-0.1610,0.2427,0.0162,-0.068092222,1.654408737,120.396603583,0.3975,0.2927,0.5071,0.1072,0.0917,0.0748,0.1480,0.1497,5.0248,0f000001,0*be15312d\n\t", "INSPVAXA,USB3,0,49.5,FINESTEERING,2107,282097.950,02000000,471d,15824;INS_ALIGNMENT_COMPLETE,INS_RTKFIXED,37.37096903981,126.72368439114,8.5953,22.3000,-0.1607,0.2384,0.0184,-0.045725766,1.917999330,120.611516024,0.3975,0.2927,0.5071,0.1072,0.0917,0.0748,0.1480,0.1497,5.0248,0f000001,0*a51c9b7d\n\t", "INSPVAXA,USB3,0,45.5,FINESTEERING,2107,282098.950,02000000,471d,15824;INS_ALIGNMENT_COMPLETE,INS_RTKFIXED,37.37096763192,126.72368689204,8.6086,22.3000,-0.1625,0.2437,0.0135,0.032441913,2.356888954,120.959811590,0.3979,0.2928,0.5071,0.1076,0.0919,0.0749,0.1479,0.1497,5.0261,0f000001,0*4f4ceb13\n\t", "INSPVAXA,USB3,0,49.5,FINESTEERING,2107,282099.450,02000000,471d,15824;INS_ALIGNMENT_COMPLETE,INS_RTKFIXED,37.37096691868,126.72368816492,8.6172,22.3000,-0.1639,0.2543,0.0151,0.021335732,2.482431048,120.995881908,0.3986,0.2930,0.5071,0.1077,0.0920,0.0749,0.1479,0.1497,5.0261,0f000001,0*203ab1e7\n\t", "INSPVAXA,USB3,0,48.5,FINESTEERING,2107,282100.450,02000000,471d,15824;INS_ALIGNMENT_COMPLETE,INS_RTKFIXED,37.37096543026,126.72369088215,8.6324,22.3000,-0.1596,0.2535,0.0180,-0.228914974,2.462239886,121.044086589,0.3992,0.2932,0.5070,0.1074,0.0920,0.0749,0.1478,0.1497,5.0245,0f000001,0*852ce3c8\n\t", "INSPVAXA,USB3,0,48.5,FINESTEERING,2107,282101.450,02000000,471d,15824;INS_ALIGNMENT_COMPLETE,INS_RTKFIXED,37.37096396393,126.72369353310,8.6472,22.3000,-0.1601,0.2590,0.0331,-0.375730399,2.404420745,120.887856332,0.3993,0.2932,0.5070,0.1073,0.0921,0.0749,0.1478,0.1497,5.0225,0f000001,0*bfa232fa\n\t", "INSPVAXA,USB3,0,48.5,FINESTEERING,2107,282101.950,02000000,471d,15824;INS_ALIGNMENT_COMPLETE,INS_RTKFIXED,37.37096322042,126.72369488771,8.6547,22.3000,-0.1481,0.2477,0.0237,-0.389461163,2.309809886,120.810766279,0.3993,0.2932,0.5070,0.1073,0.0921,0.0749,0.1478,0.1497,5.0225,0f000001,0*6153e896\n\t", "INSPVAXA,USB3,0,49.0,FINESTEERING,2107,282102.450,02000000,471d,15824;INS_ALIGNMENT_COMPLETE,INS_RTKFIXED,37.37096250169,126.72369619027,8.6639,22.3000,-0.1489,0.2563,0.0130,-0.492163713,2.419406589,120.611003212,0.3993,0.2933,0.5071,0.1074,0.0920,0.0750,0.1477,0.1497,5.0208,0f000001,0*e05fb414\n\t", "INSPVAXA,USB3,0,48.0,FINESTEERING,2107,282103.450,02000000,471d,15824;INS_ALIGNMENT_COMPLETE,INS_RTKFIXED,37.37096107043,126.72369881469,8.6799,22.3000,-0.1515,0.2464,0.0161,-0.632214670,2.279605302,119.849217483,0.3987,0.2933,0.5070,0.1074,0.0919,0.0750,0.1477,0.1496,5.0198,0f000001,0*6937ebdf\n\t", "INSPVAXA,USB3,0,48.0,FINESTEERING,2107,282103.950,02000000,471d,15824;INS_ALIGNMENT_COMPLETE,INS_RTKFIXED,37.37096036868,126.72370013653,8.6871,22.3000,-0.1575,0.2589,0.0105,-0.654965862,2.296906334,119.467685028,0.3987,0.2933,0.5070,0.1074,0.0919,0.0750,0.1477,0.1496,5.0198,0f000001,0*9d5844ee\n\t", "INSPVAXA,USB3,0,48.5,FINESTEERING,2107,282104.950,02000000,471d,15824;INS_ALIGNMENT_COMPLETE,INS_RTKFIXED,37.37095896763,126.72370277535,8.6981,22.3000,-0.1486,0.2458,0.0269,-0.592987818,1.965751442,118.674591406,0.3980,0.2932,0.5070,0.1074,0.0918,0.0751,0.1476,0.1496,5.0196,0f000001,0*607cbc7a\n\t", "INSPVAXA,USB3,0,48.5,FINESTEERING,2107,282105.450,02000000,471d,15824;INS_ALIGNMENT_COMPLETE,INS_RTKFIXED,37.37095828575,126.72370408394,8.7035,22.3000,-0.1486,0.2405,0.0183,-0.703477485,1.966758993,118.307014299,0.3974,0.2931,0.5072,0.1076,0.0917,0.0751,0.1476,0.1496,5.0199,0f000001,0*e468851e\n\t", "INSPVAXA,USB3,0,48.5,FINESTEERING,2107,282105.950,02000000,471d,15824;INS_ALIGNMENT_COMPLETE,INS_RTKFIXED,37.37095759805,126.72370541666,8.7095,22.3000,-0.1479,0.2589,0.0183,-0.776033189,1.928048544,118.044505224,0.3974,0.2931,0.5072,0.1076,0.0917,0.0751,0.1476,0.1496,5.0199,0f000001,0*d471bf4f\n\t", "INSPVAXA,USB3,0,46.5,FINESTEERING,2107,282106.450,02000000,471d,15824;INS_ALIGNMENT_COMPLETE,INS_RTKFIXED,37.37095690919,126.72370675668,8.7141,22.3000,-0.1377,0.2446,0.0099,-0.892542340,1.922749493,117.853154377,0.3968,0.2930,0.5072,0.1078,0.0917,0.0751,0.1476,0.1496,5.0204,0f000001,0*bc0c1e21\n\t", "INSPVAXA,USB3,0,46.5,FINESTEERING,2107,282106.950,02000000,471d,15824;INS_ALIGNMENT_COMPLETE,INS_RTKFIXED,37.37095621502,126.72370811365,8.7176,22.3000,-0.1440,0.2520,0.0136,-0.957648564,1.997661807,117.680291492,
